vi "ExtCall.vi"(8 "error in (no error)":errorcluster, 9 "Val":variant, 10 "Tag":u16, 11 "Pulse in":refnum<class "Rigol DG822 Pulse.lvclass">) -> (0 "error out":errorcluster, 1 "Response":variant, 3 "Pulse out":refnum<class "Rigol DG822 Pulse.lvclass">)   [LabVIEW 2021, in "Rigol DG822 UI.lvlib" / "Rigol DG822 Pulse.lvlib" / "Rigol DG822 Pulse.lvclass"]
uses:
  Rigol DG822 Pulse.lvclass
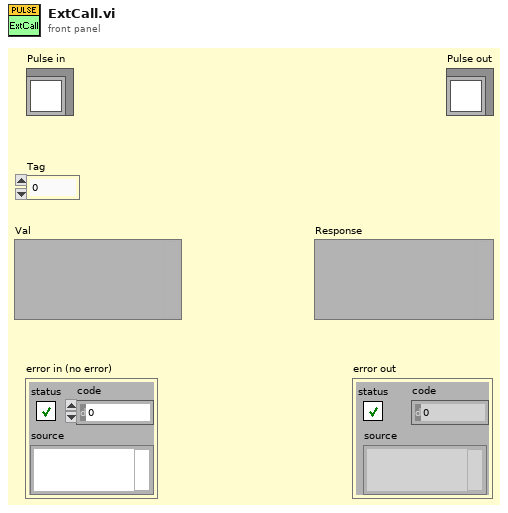
[diagram p1: front panel]
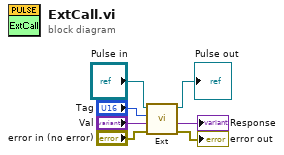
[diagram p0: block diagram]
diagram:
  n1 = call "Ext.vi"("error in (no error)"="error in (no error)", "Val"="Val", "Tag"="Tag", "Pulse in"="Pulse in") -> ("error out"=→"error out":errorcluster, "Parsed"=→"Response":variant, "Pulse out"=→"Pulse out":refnum<class "Rigol DG822 Pulse.lvclass">)  [unwired: 5 in]
